vi "exitingState.vi"(7 "statemachine":refnum<class "statemachine.lvclass">, 8 "error in (no error)":errorcluster, 10 "State Data in":refnum<class "data.lvclass">, 11 "State in":refnum<class "state.lvclass">) -> (0 "error out":errorcluster, 2 "State Data out":refnum<class "data.lvclass">, 3 "State out":refnum<class "state.lvclass">)   [LabVIEW 2020, in "eos.lvlib" / "state.lvclass"]
uses:
  state.lvclass
  data/data.lvclass
  classes/statemachine/statemachine.lvclass
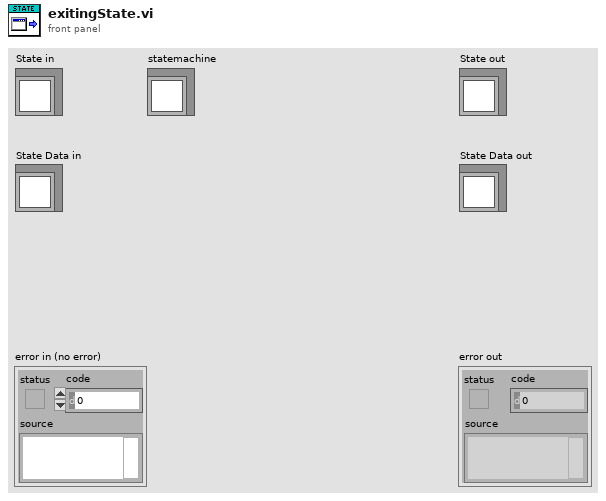
[diagram p1: front panel]
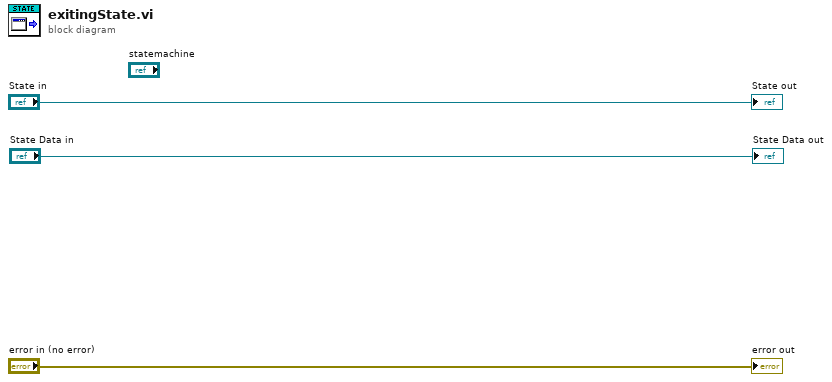
[diagram p0: block diagram]
diagram:
  "error out" <- "error in (no error)"
  "State out" <- "State in"
  "State Data out" <- "State Data in"
